vi "ParseCounterArrayToCounterMonitor.vi"(9 "MachineID":string, 11 "CountersConfigArray":T3(array[cluster])) -> (3 "CounterMonitorArray":T1(array[cluster]))   [LabVIEW 2017]
panel:
  out "UDT_1":T2
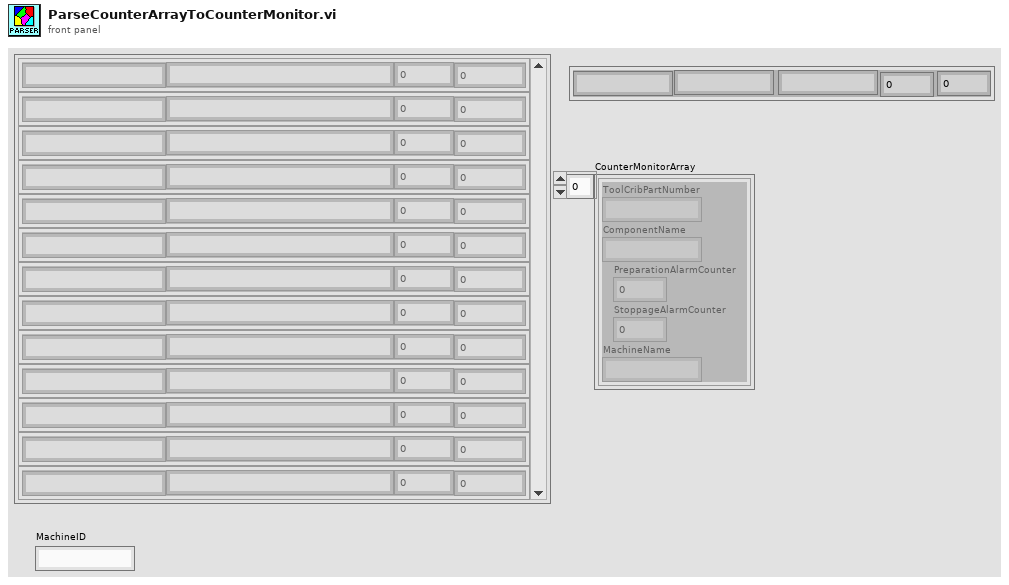
[diagram p1: front panel]
types:
  T1 = cluster{"ToolCribPartNumber":string, "ComponentName":string, "PreparationAlarmCounter":dbl, "StoppageAlarmCounter":dbl, "MachineName":string}[]
  T2 = cluster{"ToolCribPartNumber":string, "ComponentName":string, "PreparationAlarmCounter":dbl, "StoppageAlarmCounter":dbl, "MachineName":string}
  T3 = cluster{"ToolCribPartNumber":string, "ComponentName":string, "PreparationAlarmCounter":dbl, "StoppageAlarmCounter":dbl}[]
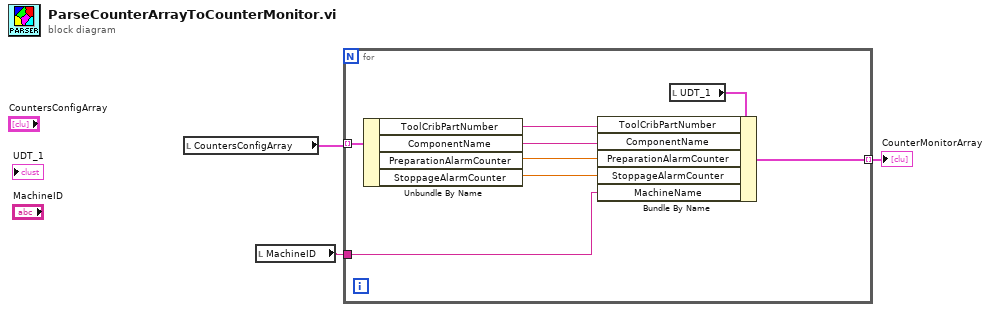
[diagram p0: block diagram]
diagram:
  n1 = local read "CountersConfigArray"() -> (w3:T3)
  n2 = local read "MachineID"() -> (w2:string)
  n3 = for {
    tunnel: w3 -> [w11] mode=indexing
    tunnel: w2 -> [w9]
    tunnel: [w4] -> w1 mode=indexing
    n4 = Unbundle By Name(w11) -> ("ToolCribPartNumber"=w8:string, "ComponentName"=w7:string, "PreparationAlarmCounter"=w6:dbl, "StoppageAlarmCounter"=w5:dbl)
    n5 = local read "UDT_1"() -> (w10:T2)
    n6 = Bundle By Name(cluster=w10, "ToolCribPartNumber"=w8, "ComponentName"=w7, "PreparationAlarmCounter"=w6, "StoppageAlarmCounter"=w5, "MachineName"=w9) -> (w4:T2)
  }
  "CounterMonitorArray" <- w1
